vi "NameJSONtoPersonnelJSON.vi"(8 "error in (no error)":errorcluster, 11 "Name JSON":string) -> (0 "error out":errorcluster, 3 "Personnel JSON":string)   [LabVIEW 2015]
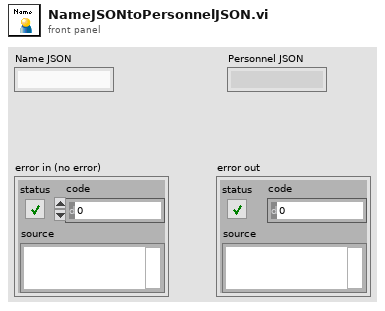
[diagram p1: front panel]
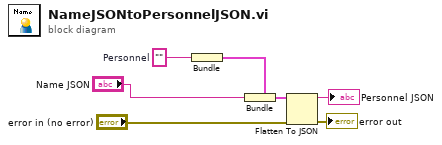
[diagram p0: block diagram]
diagram:
  w4 = ""  # Personnel
  n1 = Bundle("Personnel"=w4) -> (w5:cluster{"Personnel":string})  [unwired: 1 in]
  n2 = Bundle(cluster=w5, "Personnel"="Name JSON") -> (w6:cluster{"Personnel":string})
  n3 = Flatten To JSON(anything=w6, error in (no error)="error in (no error)") -> (JSON string=→"Personnel JSON":string, 11:→"error out":errorcluster)  [unwired: 1 in]
